vi "RecordDuringSaveSample_modified.vi"() -> ()   [LabVIEW 2015]
panel:
  out "Status":string
  out "Mem Frame Info":T1={"Start"=0, "End"=0, "Trigger"=0, "TwoStageLowToHigh"=0, "TwoStageHighToLow"=0, "TwoStageTiming"=0, "Event"=[1, 1, 1, 1, 1, 1, 1, 1, 1, 1], "EventCount"=0, "RecordedFrames"=0} {"RecordedFrames" max=0; "EventCount" max=0}
  out "IsSaving":bool
  in  "Save File Name":string caption="Save File Name :"
  in  "Save Path Name":path caption="Save Path Name :"
  out "Information":T2 caption="Frame"
  out "IsRecording":bool
  in  "Command":bool
  out "Picture":picture
  out "ChildNo":u32=1
  out "DeviceNo":u32
  in  "Stop":bool
  out "Error_Out":T3
  out "Color Type":enum16{"MONO", "COLOR"}(ring)
  out "Resolution":cluster{"Width":u32, "Height":u32}
  # "_1.avi"
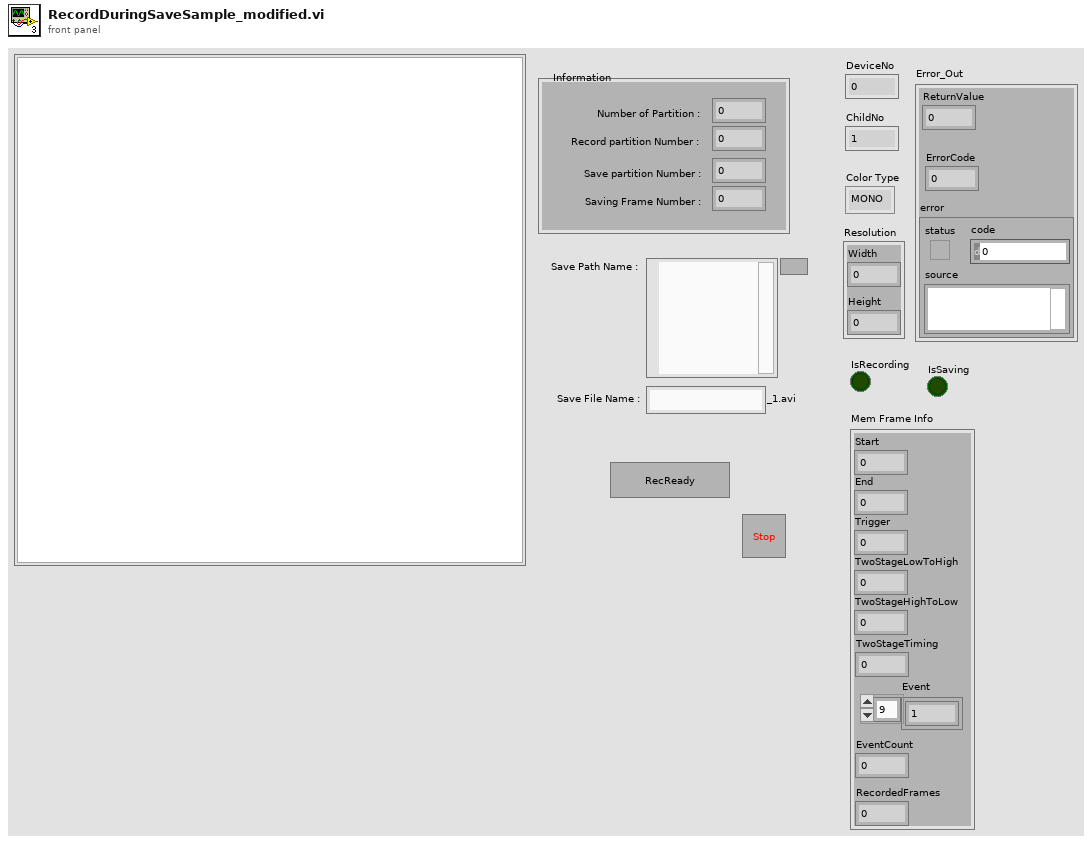
[diagram p1: front panel]
types:
  T1 = cluster{"Start":i32, "End":i32, "Trigger":i32, "TwoStageLowToHigh":i32, "TwoStageHighToLow":i32, "TwoStageTiming":u32, "Event":i32[], "EventCount":u32, "RecordedFrames":u32}
  T2 = cluster{"Number of Partition":u32, "Save Partition Number":u32, "Record Partition Number":u32, "Saving Frame Number":i32}
  T3 = cluster{"ReturnValue":u32, "ErrorCode":u32, "error ":errorcluster}
  T4 = enum16{"Initialize", "Device Initialize", "Status Check", "Save Image Open", "Save Image", "Save Image Close", "Update Window", "Default", "Exit", "Error"}
  T5 = typedef "LVBoundsTypeDef.ctl" = cluster{"Width":u32, "Height":u32}
  T6 = cluster{"Number of Partition":u32, "Save Partition Number":u32, "t":u32, "Saving Frame Number":i32}
  T7 = cluster{"Number of Partition":u32, "Save Partition Number":u32, "Record Partition Number":u32, i32}
  T8 = cluster{"Number of Partition":u32, "t":u32, "Record Partition Number":u32, "Saving Frame Number":i32}
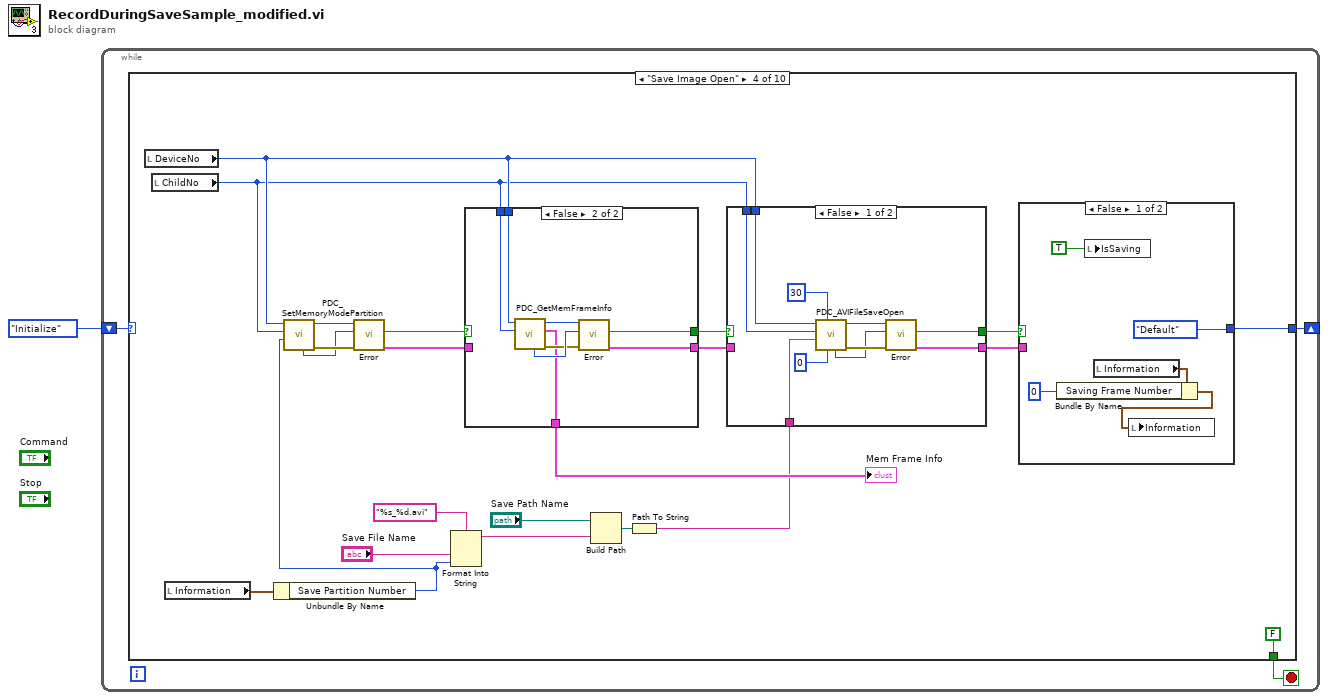
[diagram p0: block diagram]
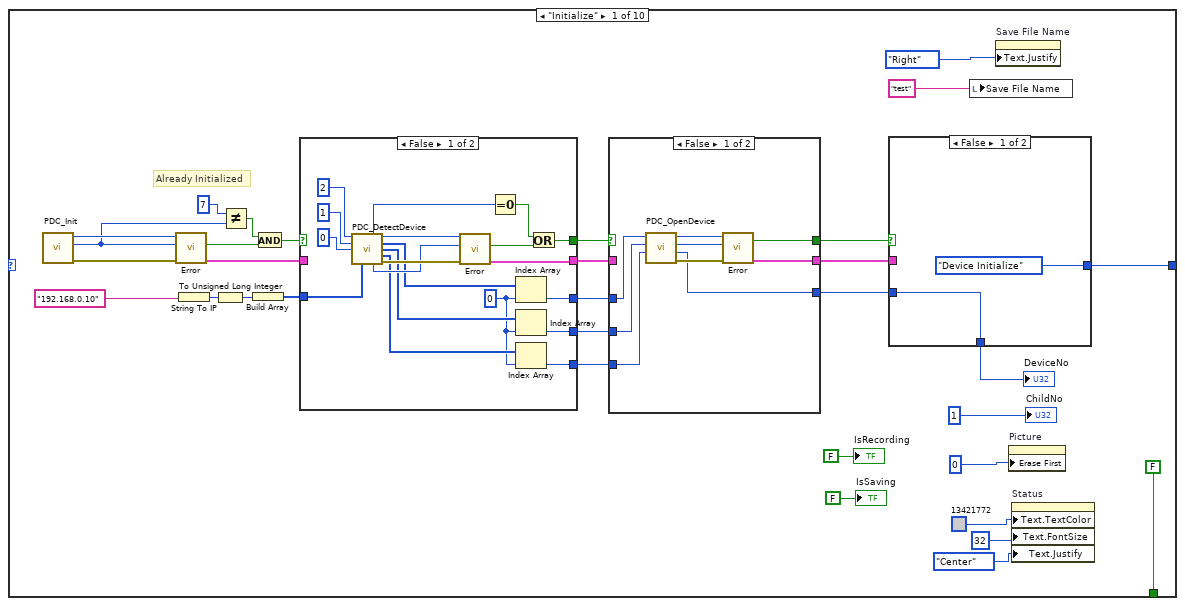
[diagram p2: hidden frame]
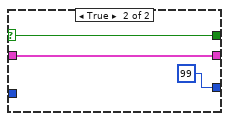
[diagram p3: hidden frame]
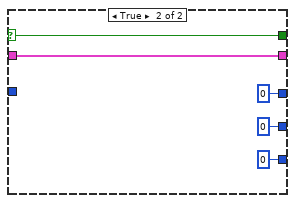
[diagram p4: hidden frame]
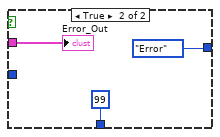
[diagram p5: hidden frame]
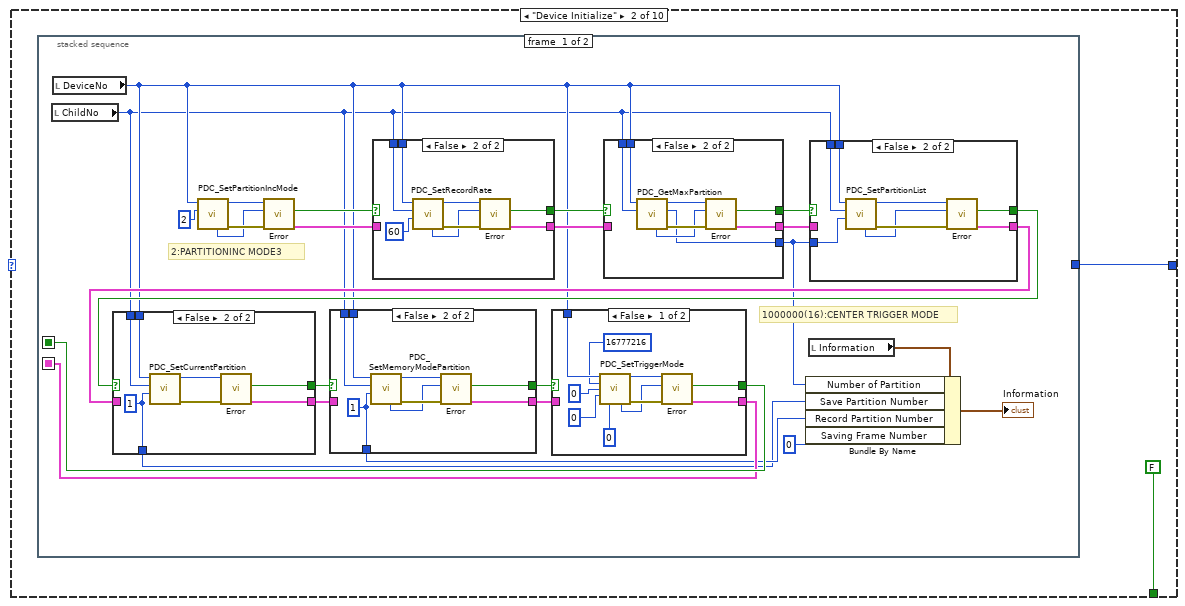
[diagram p6: hidden frame]
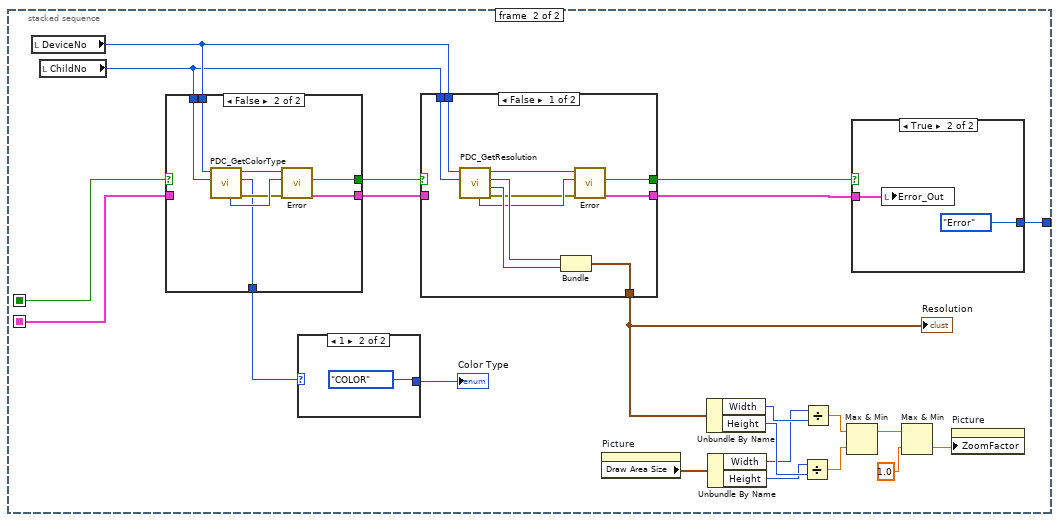
[diagram p13: hidden frame]
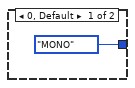
[diagram p16: hidden frame]
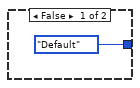
[diagram p17: hidden frame]
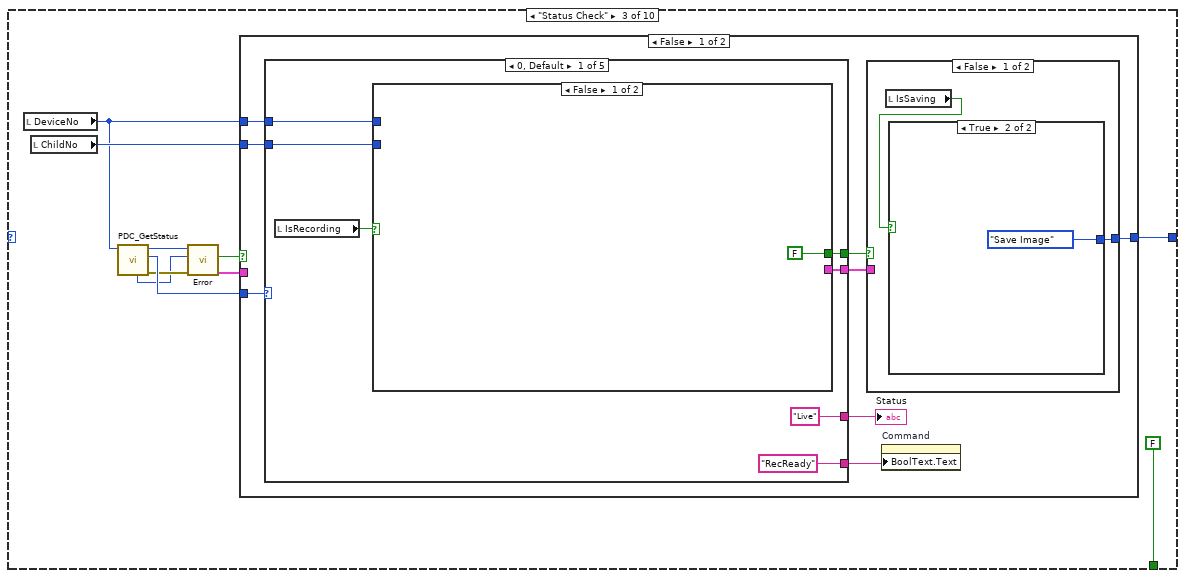
[diagram p18: hidden frame]
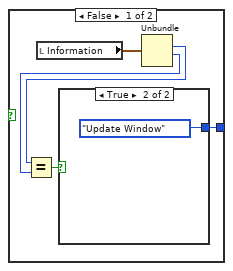
[diagram p19: hidden frame]
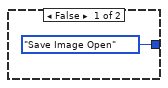
[diagram p20: hidden frame]
diagram:
  n1 = while {
    shift-right: [w2] -> _
    shift-left: T4."Initialize" ("Mode") -> [w3]
    stop <- w4 stop-if-true
    n2 = case shown="\"Save Image Open\"" w3 {
      tunnel: [FALSE FALSE FALSE FALSE FALSE FALSE FALSE FALSE TRUE FALSE] -> w4
      tunnel: [w15 w78 w216 w299 w343 w378 w405 w438 _ T4."Exit" ("Mode")] -> w2
      frame "Initialize" {
        # "Already Initialized"
        n3 = call "PDC_Init.vi"() -> ("error out"=w36:errorcluster, "ErrorCode"=w32:u32, "ReturnValue"=w35:u32)  [unwired: 9 in]
        n4 = call "Error.vi"("error in (no error)"=w36, "ErrorCode"=w32, "ReturnValue"=w35) -> ("Error_Out"=w29:T3, "Error?"=w34:bool)  [unwired: 7 in]
        n5 = String To IP(1:"192.168.0.10") -> (0:w22:u32)
        n6 = To Unsigned Long Integer(number=w22) -> (unsigned 32bit integer=w23:u32)
        n7 = Not Equal?(x=u32 7, y=w32) -> (x != y?=w33:bool)
        n8 = Build Array(w23) -> (w20:u32[])
        n9 = And(x=w33, y=w34) -> (x .and. y?=w30:bool)
        n10 = case shown="False" w30 {
          selector: w30 -> [_ w71]
          tunnel: w29 -> [_ w72]
          tunnel: [w59 w72] -> w27
          tunnel: [w61 w71] -> w28
          tunnel: w20 -> [w56 _]
          tunnel: [w51 u32 0 ("m_nDeviceCode")] -> w19
          tunnel: [w50 u32 0 ("m_nTmpDeviceNo")] -> w18
          tunnel: [w49 u32 0] -> w17
          frame False {
            w52 = 0 ("指標")
            n11 = call "PDC_DetectDevice.vi"("InterfaceCode"=u32 2, "DetectNum"=u32 1, "DetectParam"=u32 0, "DetectNo"=w56) -> ("DeviceNum"=w57:u32, "ReturnValue"=w63:u32, "DeviceCode"=w55:u32[], "TmpDeviceNo"=w54:u32[], "InterfaceCode(out)"=w53:u32[], "ErrorCode"=w62:u32, "error out"=w64:errorcluster)  [unwired: 5 in]
            n12 = call "Error.vi"("error in (no error)"=w64, "ErrorCode"=w62, "ReturnValue"=w63) -> ("Error_Out"=w59:T3, "Error?"=w60:bool)  [unwired: 7 in]
            n13 = Equal To 0?(x=w57) -> (x = 0?=w58:bool)
            n14 = Index Array(array=w55, index=w52) -> (element=w51:u32)
            n15 = Index Array(array=w54, index=w52) -> (element=w50:u32)
            n16 = Index Array(array=w53, index=w52) -> (element=w49:u32)
            n17 = Or(x=w58, y=w60) -> (x .or. y?=w61:bool)
          }
          frame True {
          }
        }
        n18 = case shown="False" w28 {
          selector: w28 -> [_ w47]
          tunnel: w27 -> [_ w48]
          tunnel: [w45 w48] -> w24
          tunnel: [w38 w47] -> w25
          tunnel: w19 -> [w39 _]
          tunnel: w18 -> [w40 _]
          tunnel: w17 -> [w41 _]
          tunnel: [w37 u32 99 ("DeviceNo")] -> w16
          frame False {
            n19 = call "PDC_OpenDevice.vi"("InterfaceCode"=w41, "TmpDeviceNo"=w40, "DeviceCode"=w39) -> ("error out"=w44:errorcluster, "DeviceNo"=w37:u32, "ErrorCode"=w42:u32, "ReturnValue"=w43:u32)  [unwired: 5 in]
            n20 = call "Error.vi"("error in (no error)"=w44, "ErrorCode"=w42, "ReturnValue"=w43) -> ("Error_Out"=w45:T3, "Error?"=w38:bool)  [unwired: 7 in]
          }
          frame True {
          }
        }
        n21 = case shown="False" w25 {
          tunnel: [T4."Device Initialize" ("Mode") T4."Error" ("Mode")] -> w15
          tunnel: w24 -> [_ w76]
          tunnel: w16 -> [w74 _]
          tunnel: [w74 u32 99 ("DeviceNo")] -> w12
          frame False {
          }
          frame True {
            "Error_Out" <- w76
          }
        }
        "DeviceNo" <- w12
        n22 = local write "Save File Name"("test" ("Save File Name")) -> ()
        n23 = property on="Save File Name" class="Str"("Text.Justify"=enum16{"Left", "Center", "Right"}."Right" ("テキスト.位置調整")) -> ()  [unwired: 2 in, 2 out]
        n24 = property on="Picture" class="Pict"("Erase First"=u8 0 ("最初に削除")) -> ()  [unwired: 2 in, 2 out]
        n25 = property on="Status" class="Str"("Text.TextColor"=u32 13421772, "Text.FontSize"=u32 32 ("テキスト.フォント:サイズ"), "Text.Justify"=enum16{"Left", "Center", "Right"}."Center" ("テキスト.位置調整")) -> ()  [unwired: 2 in, 2 out]
        "IsRecording" <- FALSE ("IsRecord")
        "ChildNo" <- u32 1
        "IsSaving" <- FALSE ("IsRecord")
      }
      frame "Device Initialize" {
        n26 = stacked-sequence {
          seq-local: [w88 _] -> [_ w181]
          seq-local: [w89 _] -> [_ w182]
          tunnel: [_ w178] -> w78
          frame #0 {
            # "1000000(16):CENTER TRIGGER MODE"
            # "2:PARTITIONINC MODE3"
            n27 = local read "ChildNo"() -> (w86:u32)
            n28 = local read "DeviceNo"() -> (w87:u32)
            n29 = call "PDC_SetPartitionIncMode.vi"("Mode"=u32 2, "DeviceNo"=w87) -> ("error out"=w104:errorcluster, "ReturnValue"=w105:u32, "ErrorCode"=w103:u32)  [unwired: 7 in]
            n30 = call "Error.vi"("error in (no error)"=w104, "ErrorCode"=w103, "ReturnValue"=w105) -> ("Error_Out"=w100:T3, "Error?"=w101:bool)  [unwired: 7 in]
            n31 = case shown="False" w101 {
              selector: w101 -> [w158 _]
              tunnel: w100 -> [w157 _]
              tunnel: [w157 w163] -> w99
              tunnel: [w158 w162] -> w98
              tunnel: w87 -> [_ w161]
              tunnel: w86 -> [_ w160]
              frame True {
              }
              frame False {
                n32 = call "PDC_SetRecordRate.vi"("Rate"=u32 60, "ChildNo"=w160, "DeviceNo"=w161) -> ("error out"=w165:errorcluster, "ReturnValue"=w166:u32, "ErrorCode"=w164:u32)  [unwired: 6 in]
                n33 = call "Error.vi"("error in (no error)"=w165, "ErrorCode"=w164, "ReturnValue"=w166) -> ("Error_Out"=w163:T3, "Error?"=w162:bool)  [unwired: 7 in]
              }
            }
            n34 = case shown="False" w98 {
              selector: w98 -> [w148 _]
              tunnel: w99 -> [w147 _]
              tunnel: [w148 w154] -> w97
              tunnel: [w147 w153] -> w96
              tunnel: w87 -> [_ w151]
              tunnel: w86 -> [_ w150]
              tunnel: [_ w149] -> w83
              frame True {
              }
              frame False {
                n35 = call "PDC_GetMaxPartition.vi"("ChildNo"=w150, "DeviceNo"=w151) -> ("error out"=w155:errorcluster, "Count"=w149:u32, "ReturnValue"=w156:u32, "ErrorCode"=w152:u32)  [unwired: 5 in, 1 out]
                n36 = call "Error.vi"("error in (no error)"=w155, "ErrorCode"=w152, "ReturnValue"=w156) -> ("Error_Out"=w153:T3, "Error?"=w154:bool)  [unwired: 7 in]
              }
            }
            n37 = local read "Information"() -> (w85:T2)
            n38 = case shown="False" w97 {
              selector: w97 -> [w138 _]
              tunnel: w96 -> [w137 _]
              tunnel: [w138 w143] -> w93
              tunnel: [w137 w142] -> w92
              tunnel: w87 -> [_ w141]
              tunnel: w86 -> [_ w140]
              tunnel: w83 -> [_ w139]
              frame True {
              }
              frame False {
                n39 = call "PDC_SetPartitionList.vi"("Count"=w139, "ChildNo"=w140, "DeviceNo"=w141) -> ("error out"=w146:errorcluster, "ReturnValue"=w145:u32, "ErrorCode"=w144:u32)  [unwired: 6 in]
                n40 = call "Error.vi"("error in (no error)"=w146, "ErrorCode"=w144, "ReturnValue"=w145) -> ("Error_Out"=w142:T3, "Error?"=w143:bool)  [unwired: 7 in]
              }
            }
            n41 = case shown="False" w93 {
              selector: w93 -> [w129 _]
              tunnel: [w129 w134] -> w95
              tunnel: [w128 w133] -> w94
              tunnel: w92 -> [w128 _]
              tunnel: w87 -> [_ w132]
              tunnel: w86 -> [_ w131]
              tunnel: [_ w130] -> w80
              frame True {
              }
              frame False {
                w130 = u32 1 ("No")
                n42 = call "PDC_SetCurrentPartition.vi"("No"=w130, "ChildNo"=w131, "DeviceNo"=w132) -> ("error out"=w135:errorcluster, "ReturnValue"=w136:u32)  [unwired: 6 in, 1 out]
                n43 = call "Error.vi"("error in (no error)"=w135, "ReturnValue"=w136) -> ("Error_Out"=w133:T3, "Error?"=w134:bool)  [unwired: 8 in]
              }
            }
            n44 = case shown="False" w95 {
              selector: w95 -> [w119 _]
              tunnel: w94 -> [w118 _]
              tunnel: [w119 w124] -> w91
              tunnel: [w118 w121] -> w90
              tunnel: w87 -> [_ w123]
              tunnel: w86 -> [_ w122]
              tunnel: [_ w120] -> w81
              frame True {
              }
              frame False {
                w120 = u32 1 ("No")
                n45 = call "PDC_SetMemoryModePartition.vi"("No"=w120, "ChildNo"=w122, "DeviceNo"=w123) -> ("error out"=w126:errorcluster, "ReturnValue"=w127:u32, "ErrorCode"=w125:u32)  [unwired: 6 in]
                n46 = call "Error.vi"("error in (no error)"=w126, "ErrorCode"=w125, "ReturnValue"=w127) -> ("Error_Out"=w121:T3, "Error?"=w124:bool)  [unwired: 7 in]
              }
            }
            n47 = case shown="False" w91 {
              selector: w91 -> [_ w117]
              tunnel: w90 -> [_ w116]
              tunnel: [w111 w117] -> w89
              tunnel: [w115 w116] -> w88
              tunnel: w87 -> [w110 _]
              frame False {
                n48 = call "PDC_SetTriggerMode.vi"("DeviceNo"=w110, "Mode"=u32 16777216, "AFrames"=u32 0, "RFrames"=u32 0, "RCount"=u32 0) -> ("ReturnValue"=w113:u32, "ErrorCode"=w112:u32, "error out"=w114:errorcluster)  [unwired: 8 in]
                n49 = call "Error.vi"("error in (no error)"=w114, "ErrorCode"=w112, "ReturnValue"=w113) -> ("Error_Out"=w115:T3, "Error?"=w111:bool)  [unwired: 7 in]
              }
              frame True {
              }
            }
            n50 = Bundle By Name(cluster=w85, "Number of Partition"=w83, "Save Partition Number"=w80, "Record Partition Number"=w81, "Saving Frame Number"=0) -> (→"Information":T2)
          }
          frame #1 {
            n51 = local read "DeviceNo"() -> (w180:u32)
            n52 = local read "ChildNo"() -> (w179:u32)
            n53 = case shown="False" w182 {
              selector: w182 -> [w190 _]
              tunnel: [_ w195] -> w188
              tunnel: [w190 w194] -> w186
              tunnel: [w189 w193] -> w185
              tunnel: w181 -> [w189 _]
              tunnel: w180 -> [_ w192]
              tunnel: w179 -> [_ w191]
              frame True {
              }
              frame False {
                n54 = call "PDC_GetColorType.vi"("ChildNo"=w191, "DeviceNo"=w192) -> ("error out"=w196:errorcluster, "Mode"=w195:i8, "ReturnValue"=w198:u32, "ErrorCode"=w197:u32)  [unwired: 6 in]
                n55 = call "Error.vi"("error in (no error)"=w196, "ErrorCode"=w197, "ReturnValue"=w198) -> ("Error_Out"=w193:T3, "Error?"=w194:bool)  [unwired: 7 in]
              }
            }
            n56 = case shown="1" w188 {
              tunnel: [enum16{"MONO", "COLOR"}."MONO" enum16{"MONO", "COLOR"}."COLOR"] -> w187
              frame 0, Default {
              }
              frame 1 {
              }
            }
            "Color Type" <- w187
            n57 = case shown="False" w186 {
              selector: w186 -> [_ w209]
              tunnel: w185 -> [_ w210]
              tunnel: [w202 w210] -> w183
              tunnel: [w203 w209] -> w184
              tunnel: [w201 _] -> w176
              tunnel: w180 -> [w200 _]
              tunnel: w179 -> [w199 _]
              frame False {
                n58 = call "PDC_GetResolution.vi"("ChildNo"=w199, "DeviceNo"=w200) -> ("error out"=w205:errorcluster, "Height"=w208:u32, "Width"=w207:u32, "ReturnValue"=w204:u32, "ErrorCode"=w206:u32)  [unwired: 5 in]
                n59 = Bundle("Width"=w207, "Height"=w208) -> (w201:cluster{"Width":u32, "Height":u32})  [unwired: 1 in]
                n60 = call "Error.vi"("error in (no error)"=w205, "ErrorCode"=w206, "ReturnValue"=w204) -> ("Error_Out"=w202:T3, "Error?"=w203:bool)  [unwired: 7 in]
              }
              frame True {
              }
            }
            "Resolution" <- w176
            n61 = property on="Picture" class="Pict"() -> ("Draw Area Size"=w177:T5)  [unwired: 2 in, 2 out]
            n62 = Unbundle By Name(w176) -> ("Width"=w175:u32, "Height"=w174:u32)
            n63 = Unbundle By Name(w177) -> ("Width"=w173:u32, "Height"=w172:u32)
            n64 = Divide(x=w172, y=w174) -> (x/y=w170:dbl)
            n65 = Divide(x=w173, y=w175) -> (x/y=w171:dbl)
            n66 = Max & Min(x=w171, y=w170) -> (max(x,y)=w169:dbl)  [unwired: 1 out]
            n67 = case shown="True" w184 {
              tunnel: [T4."Default" ("Mode") T4."Error" ("Mode")] -> w178
              tunnel: w183 -> [_ w215]
              frame False {
              }
              frame True {
                n68 = local write "Error_Out"(w215) -> ()
              }
            }
            n69 = Max & Min(x=w169, y=1.0) -> (min(x,y)=w168:dbl)  [unwired: 1 out]
            n70 = property on="Picture" class="Pict"("ZoomFactor"=w168) -> ()  [unwired: 2 in, 2 out]
          }
        }
      }
      frame "Status Check" {
        n71 = local read "DeviceNo"() -> (w220:u32)
        n72 = local read "ChildNo"() -> (w221:u32)
        n73 = call "PDC_GetStatus.vi"("DeviceNo"=w220) -> ("error out"=w219:errorcluster, "Status"=w222:u32, "ReturnValue"=w218:u32, "ErrorCode"=w217:u32)  [unwired: 7 in]
        n74 = call "Error.vi"("error in (no error)"=w219, "ErrorCode"=w217, "ReturnValue"=w218) -> ("Error_Out"=w223:T3, "Error?"=w224:bool)  [unwired: 7 in]
        n75 = case shown="False" w224 {
          tunnel: w223 -> [_ w281]
          tunnel: w222 -> [w233 _]
          tunnel: w220 -> [w232 _]
          tunnel: w221 -> [w231 _]
          tunnel: [w227 T4."Error" ("Mode")] -> w216
          frame False {
            n76 = case shown="0, Default" w233 {
              tunnel: w232 -> [w251 _ _ _ _]
              tunnel: w231 -> [w250 _ _ _ _]
              tunnel: ["Live" "PlayBack" "RecReady" "Endless" "Record"] -> w226
              tunnel: ["RecReady" "Live" "Trigger In" "Trigger In" "Cancel"] -> w230
              tunnel: [w247 _ _ _ _] -> w229
              tunnel: [w246 _ _ _ _] -> w228
              frame 0, Default {
                n77 = local read "IsRecording"() -> (w252:bool)
                n78 = case shown="False" w252 {
                  tunnel: w251 -> [_ w259]
                  tunnel: w250 -> [_ w258]
                  tunnel: [FALSE ("Error?") w257] -> w247
                  tunnel: [_ w256] -> w246
                  frame False {
                  }
                  frame True {
                    n79 = local read "Information"() -> (w267:T2)
                    n80 = local write "IsRecording"(FALSE ("IsRecord")) -> ()
                    n81 = Unbundle(w267) -> ("Number of Partition"=w263:u32, "Save Partition Number"=w255:u32, "Record Partition Number"=w266:u32, "Saving Frame Number"=w264:i32)
                    n82 = Equal?(x=w263, y=w266) -> (x = y?=w270:bool)
                    n83 = Increment(x=w266) -> (x+1=w268:u32)
                    n84 = Select(t=u32 1, s=w270, f=w268) -> (s? t:f=w254:u32)
                    n85 = call "PDC_SetCurrentPartition.vi"("No"=w254, "ChildNo"=w258, "DeviceNo"=w259) -> ("error out"=w262:errorcluster, "ReturnValue"=w261:u32, "ErrorCode"=w260:u32)  [unwired: 6 in]
                    n86 = call "Error.vi"("error in (no error)"=w262, "ErrorCode"=w260, "ReturnValue"=w261) -> ("Error_Out"=w256:T3, "Error?"=w257:bool)  [unwired: 7 in]
                    n87 = Bundle("Number of Partition"=w263, "Save Partition Number"=w255, "t"=w254, "Saving Frame Number"=w264) -> (w265:T6)  [unwired: 1 in]
                    n88 = local write "Information"(w265) -> ()
                  }
                }
              }
              frame 1 {
              }
              frame 2 {
              }
              frame 4 {
              }
              frame 8 {
              }
            }
            "Status" <- w226
            n89 = case shown="False" w229 {
              tunnel: w228 -> [_ w245]
              tunnel: [w234 T4."Error" ("Mode")] -> w227
              frame False {
                n90 = local read "IsSaving"() -> (w235:bool)
                n91 = case shown="True" w235 {
                  tunnel: [w236 T4."Save Image" ("Mode")] -> w234
                  frame False {
                    n92 = local read "Information"() -> (w240:T2)
                    n93 = Unbundle(w240) -> ("Save Partition Number"=w237:u32, "Record Partition Number"=w238:u32)  [unwired: 2 out]
                    n94 = Equal?(x=w237, y=w238) -> (x = y?=w239:bool)
                    n95 = case shown="True" w239 {
                      tunnel: [T4."Save Image Open" ("Mode") T4."Update Window" ("Mode")] -> w236
                      frame False {
                      }
                      frame True {
                      }
                    }
                  }
                  frame True {
                  }
                }
              }
              frame True {
                n96 = local write "Error_Out"(w245) -> ()
              }
            }
            n97 = property on="Command" class="Bool (strict)"("BoolText.Text"=w230) -> ()  [unwired: 2 in, 2 out]
          }
          frame True {
            n98 = local write "Error_Out"(w281) -> ()
          }
        }
      }
      frame "Save Image Open" {
        n99 = local read "DeviceNo"() -> (w286:u32)
        n100 = local read "ChildNo"() -> (w285:u32)
        n101 = local read "Information"() -> (w292:T2)
        n102 = Unbundle By Name(w292) -> ("Save Partition Number"=w282:u32)
        n103 = call "PDC_SetMemoryModePartition.vi"("No"=w282, "ChildNo"=w285, "DeviceNo"=w286) -> ("error out"=w288:errorcluster, "ReturnValue"=w289:u32, "ErrorCode"=w287:u32)  [unwired: 6 in]
        n104 = call "Error.vi"("error in (no error)"=w288, "ErrorCode"=w287, "ReturnValue"=w289) -> ("Error_Out"=w283:T3, "Error?"=w284:bool)  [unwired: 7 in]
        n105 = Format Into String(format string="%s_%d.avi" ("形式文字列"), "Save File Name", w282) -> (resulting string=w291:string)  [unwired: 2 in, 1 out]
        n106 = case shown="False" w284 {
          selector: w284 -> [w305 _]
          tunnel: [w305 w310] -> w303
          tunnel: [w304 w309] -> w302
          tunnel: w286 -> [_ w308]
          tunnel: w285 -> [_ w307]
          tunnel: [_ w306] -> w298
          tunnel: w283 -> [w304 _]
          frame True {
          }
          frame False {
            n107 = call "PDC_GetMemFrameInfo.vi"("ChildNo"=w307, "DeviceNo"=w308) -> ("error out"=w311:errorcluster, "Frame"=w306:T1, "ReturnValue"=w312:u32, "ErrorCode"=w313:u32)  [unwired: 6 in]
            n108 = call "Error.vi"("error in (no error)"=w311, "ErrorCode"=w313, "ReturnValue"=w312) -> ("Error_Out"=w309:T3, "Error?"=w310:bool)  [unwired: 7 in]
          }
        }
        "Mem Frame Info" <- w298
        n109 = Build Path(base path="Save Path Name", name or relative path=w291) -> (appended path=w295:path)
        n110 = Path To String(path=w295) -> (string=w290:string)
        n111 = case shown="False" w303 {
          selector: w303 -> [_ w332]
          tunnel: w302 -> [_ w331]
          tunnel: [w329 w332] -> w301
          tunnel: [w330 w331] -> w300
          tunnel: w286 -> [w324 _]
          tunnel: w285 -> [w323 _]
          tunnel: w290 -> [w325 _]
          frame False {
            n112 = call "PDC_AVIFileSaveOpen.vi"("ShowCompressDlg"=u32 0, "Rate"=30, "FileName"=w325, "ChildNo"=w323, "DeviceNo"=w324) -> ("error out"=w327:errorcluster, "ReturnValue"=w328:u32, "ErrorCode"=w326:u32)  [unwired: 4 in]
            n113 = call "Error.vi"("error in (no error)"=w327, "ErrorCode"=w326, "ReturnValue"=w328) -> ("Error_Out"=w330:T3, "Error?"=w329:bool)  [unwired: 7 in]
          }
          frame True {
          }
        }
        n114 = case shown="False" w301 {
          tunnel: w300 -> [_ w320]
          tunnel: [T4."Default" ("Mode") T4."Error" ("Mode")] -> w299
          frame False {
            n115 = local write "IsSaving"(TRUE) -> ()
            n116 = local read "Information"() -> (w315:T2)
            n117 = Bundle By Name(cluster=w315, "Saving Frame Number"=0) -> (w314:T2)
            n118 = local write "Information"(w314) -> ()
          }
          frame True {
            n119 = local write "Error_Out"(w320) -> ()
          }
        }
      }
      frame "Save Image" {
        n120 = local read "Mem Frame Info"() -> (w355:T1)
        n121 = local read "Information"() -> (w356:T2)
        n122 = Unbundle(w356) -> ("Number of Partition"=w350:u32, "Save Partition Number"=w349:u32, "Record Partition Number"=w348:u32, "Saving Frame Number"=w347:i32)
        n123 = Unbundle By Name(w355) -> ("RecordedFrames"=w335:u32, "Start"=w351:i32, "End"=w352:i32)
        n124 = Add(x=w351, y=w347) -> (x+y=w354:i32)
        n125 = Increment(x=w347) -> (x+1=w334:i32)
        n126 = Less Than 0?(x=w354) -> (x < 0?=w353:bool)
        n127 = case shown="False" w353 {
          tunnel: w354 -> [w364 w367]
          tunnel: [w364 w365] -> w337
          tunnel: w352 -> [_ w368]
          tunnel: w351 -> [_ w370]
          frame False {
          }
          frame True {
            n128 = Absolute Value(x=w370) -> (abs(x)=w369:i32)
            n129 = Compound Arithmetic op=ADD(w369, w368, w367, 1 ("値")) -> (w365:i32)
          }
        }
        n130 = local read "DeviceNo"() -> (w339:u32)
        n131 = local read "ChildNo"() -> (w338:u32)
        n132 = Bundle("Number of Partition"=w350, "Save Partition Number"=w349, "Record Partition Number"=w348, w334) -> (w346:T7)  [unwired: 1 in]
        n133 = local write "Information"(w346) -> ()
        n134 = call "PDC_AVIFileSave.vi"("FrameNo"=w337, "ChildNo"=w338, "DeviceNo"=w339) -> ("error out"=w341:errorcluster, "ReturnValue"=w342:u32, "ErrorCode"=w340:u32)  [unwired: 5 in, 1 out]
        n135 = To Unsigned Long Integer(number=w334) -> (unsigned 32bit integer=w333:u32)
        n136 = call "Error.vi"("error in (no error)"=w341, "ErrorCode"=w340, "ReturnValue"=w342) -> ("Error_Out"=w344:T3, "Error?"=w345:bool)  [unwired: 7 in]
        n137 = Equal?(x=w335, y=w333) -> (x = y?=w336:bool)
        n138 = case shown="False" w345 {
          tunnel: w344 -> [_ w363]
          tunnel: [w359 T4."Save Image Close" ("Mode")] -> w343
          tunnel: w336 -> [w358 _]
          frame False {
            n139 = case shown="False" w358 {
              tunnel: [T4."Update Window" ("Mode") T4."Save Image Close" ("Mode")] -> w359
              frame False {
              }
              frame True {
              }
            }
          }
          frame True {
            n140 = local write "Error_Out"(w363) -> ()
          }
        }
      }
      frame "Save Image Close" {
        n141 = local read "DeviceNo"() -> (w372:u32)
        n142 = local read "ChildNo"() -> (w371:u32)
        n143 = call "PDC_AVIFileSaveClose.vi"("ChildNo"=w371, "DeviceNo"=w372) -> ("error out"=w375:errorcluster, "ReturnValue"=w374:u32, "ErrorCode"=w373:u32)  [unwired: 7 in]
        n144 = call "Error.vi"("error in (no error)"=w375, "ErrorCode"=w373, "ReturnValue"=w374) -> ("Error_Out"=w381:T3, "Error?"=w382:bool)  [unwired: 7 in]
        n145 = case shown="False" w382 {
          selector: w382 -> [_ w404]
          tunnel: w381 -> [_ w403]
          tunnel: [w393 w404] -> w380
          tunnel: [w392 w403] -> w379
          tunnel: w372 -> [w387 _]
          tunnel: w371 -> [w386 _]
          frame False {
            n146 = local read "Information"() -> (w402:T2)
            n147 = Unbundle(w402) -> ("Number of Partition"=w397:u32, "Save Partition Number"=w395:u32, "Record Partition Number"=w399:u32, "Saving Frame Number"=w400:i32)
            n148 = Equal?(x=w397, y=w395) -> (x = y?=w398:bool)
            n149 = Increment(x=w395) -> (x+1=w396:u32)
            n150 = Select(t=u32 1, s=w398, f=w396) -> (s? t:f=w388:u32)
            n151 = call "PDC_SetMemoryModePartition.vi"("No"=w388, "ChildNo"=w386, "DeviceNo"=w387) -> ("error out"=w390:errorcluster, "ReturnValue"=w391:u32, "ErrorCode"=w389:u32)  [unwired: 6 in]
            n152 = call "Error.vi"("error in (no error)"=w390, "ErrorCode"=w389, "ReturnValue"=w391) -> ("Error_Out"=w392:T3, "Error?"=w393:bool)  [unwired: 7 in]
            n153 = Bundle("Number of Partition"=w397, "t"=w388, "Record Partition Number"=w399, "Saving Frame Number"=w400) -> (w401:T8)  [unwired: 1 in]
            n154 = local write "Information"(w401) -> ()
          }
          frame True {
          }
        }
        n155 = case shown="False" w380 {
          tunnel: w379 -> [_ w385]
          tunnel: [T4."Default" ("Mode") T4."Error" ("Mode")] -> w378
          frame False {
          }
          frame True {
            n156 = local write "Error_Out"(w385) -> ()
          }
        }
        n157 = local write "IsSaving"(FALSE ("IsSaving")) -> ()
      }
      frame "Update Window" {
        n158 = local read "Information"() -> (w416:T2)
        n159 = Unbundle By Name(w416) -> ("Saving Frame Number"=w415:i32)
        n160 = local read "IsSaving"() -> (w412:bool)
        n161 = local read "Color Type"() -> (w409:enum16{"MONO", "COLOR"})
        n162 = local read "Resolution"() -> (w408:cluster{"Width":u32, "Height":u32})
        n163 = local read "DeviceNo"() -> (w411:u32)
        n164 = local read "ChildNo"() -> (w410:u32)
        n165 = Quotient & Remainder(x=w415, y=8) -> (x-y*floor(x/y)=w407:i32)  [unwired: 1 out]
        n166 = Not Equal To 0?(x=w407) -> (x != 0?=w406:bool)
        n167 = And(x=w412, y=w406) -> (x .and. y?=w413:bool)
        n168 = case shown="False" w413 {
          tunnel: w411 -> [_ w426]
          tunnel: w410 -> [_ w425]
          tunnel: w409 -> [_ w421]
          tunnel: w408 -> [_ w420]
          tunnel: [T4."Default" ("Mode") w422] -> w405
          frame True {
          }
          frame False {
            n169 = call "PDC_GetLiveImageData.vi"("Resolution"=w420, "ColorType"=w421, "BitDepth"=u32 8, "ChildNo"=w425, "DeviceNo"=w426) -> ("error out"=w427:errorcluster, "ErrorCode"=w429:u32, "ReturnValue"=w428:u32, "Data(8Bit)"=w419:u8[])  [unwired: 2 in, 1 out]
            n170 = call "Error.vi"("error in (no error)"=w427, "ErrorCode"=w429, "ReturnValue"=w428) -> ("Error_Out"=w423:T3, "Error?"=w424:bool)  [unwired: 7 in]
            n171 = case shown="False" w424 {
              tunnel: [T4."Error" ("Mode") T4."Default" ("Mode")] -> w422
              tunnel: w423 -> [w431 _]
              tunnel: w421 -> [_ w435]
              tunnel: w420 -> [_ w434]
              tunnel: w419 -> [_ w433]
              frame True {
                n172 = local write "Error_Out"(w431) -> ()
              }
              frame False {
                n173 = call "GetPictureData.vi"("Resolution"=w434, "Data(8Bit)"=w433, "ColorType"=w435) -> ("new picture"=→"Picture":picture)  [unwired: 4 in]
              }
            }
          }
        }
      }
      frame "Default", Default {
        n174 = event shown="[0] Timeout" {
          selector: _ -> [_ _ _]
          dyn-events: _ -> [_ _ _]
          timeout: 1 -> [_ _ _]
          tunnel: [T4."Status Check" ("Mode") w442 T4."Exit" ("Mode")] -> w438
          event Timeout {
            n175 = event-data() -> ()  [unwired: 1 in, 2 out]
          }
          event "Command": Value Change {
            n176 = event-data() -> ("NewVal"=w443:bool)  [unwired: 1 in, 4 out]
            n177 = case shown="True" w443 {
              tunnel: [T4."Default" ("Mode") w446] -> w442
              frame False {
              }
              frame True {
                n178 = local read "DeviceNo"() -> (w445:u32)
                n179 = call "PDC_GetStatus.vi"("DeviceNo"=w445) -> ("error out"=w454:errorcluster, "Status"=w449:u32, "ReturnValue"=w453:u32, "ErrorCode"=w452:u32)  [unwired: 7 in]
                n180 = call "Error.vi"("error in (no error)"=w454, "ErrorCode"=w452, "ReturnValue"=w453) -> ("Error_Out"=w450:T3, "Error?"=w451:bool)  [unwired: 7 in]
                n181 = case shown="False" w451 {
                  selector: w451 -> [_ w496]
                  tunnel: w450 -> [_ w497]
                  tunnel: [w459 w497] -> w447
                  tunnel: [w458 w496] -> w448
                  tunnel: w449 -> [w461 _]
                  tunnel: w445 -> [w460 _]
                  frame False {
                    n182 = case shown="8" w461 {
                      tunnel: w460 -> [w462 w470 w476 w483 w491]
                      tunnel: [w467 w474 w481 w488 w495] -> w459
                      tunnel: [w466 w473 w480 w487 w494] -> w458
                      frame 0, Default {
                        n183 = call "PDC_SetRecReady.vi"("DeviceNo"=w462) -> ("error out"=w465:errorcluster, "ReturnValue"=w464:u32, "ErrorCode"=w463:u32)  [unwired: 8 in]
                        n184 = call "Error.vi"("error in (no error)"=w465, "ErrorCode"=w463, "ReturnValue"=w464) -> ("Error_Out"=w467:T3, "Error?"=w466:bool)  [unwired: 7 in]
                      }
                      frame 1 {
                        n185 = call "PDC_SetStatus.vi"("Mode"=u32 0, "DeviceNo"=w470) -> ("error out"=w472:errorcluster, "ReturnValue"=w471:u32, "ErrorCode"=w469:u32)  [unwired: 7 in]
                        n186 = call "Error.vi"("error in (no error)"=w472, "ErrorCode"=w469, "ReturnValue"=w471) -> ("Error_Out"=w474:T3, "Error?"=w473:bool)  [unwired: 7 in]
                      }
                      frame 2 {
                        n187 = call "PDC_TriggerIn.vi"("DeviceNo"=w476) -> ("error out"=w479:errorcluster, "ReturnValue"=w478:u32, "ErrorCode"=w477:u32)  [unwired: 8 in]
                        n188 = call "Error.vi"("error in (no error)"=w479, "ErrorCode"=w477, "ReturnValue"=w478) -> ("Error_Out"=w481:T3, "Error?"=w480:bool)  [unwired: 7 in]
                        n189 = local write "IsRecording"(TRUE ("IsRecord")) -> ()
                      }
                      frame 4 {
                        n190 = call "PDC_TriggerIn.vi"("DeviceNo"=w483) -> ("error out"=w486:errorcluster, "ReturnValue"=w485:u32, "ErrorCode"=w484:u32)  [unwired: 8 in]
                        n191 = call "Error.vi"("error in (no error)"=w486, "ErrorCode"=w484, "ReturnValue"=w485) -> ("Error_Out"=w488:T3, "Error?"=w487:bool)  [unwired: 7 in]
                        n192 = local write "IsRecording"(TRUE ("IsRecord")) -> ()
                      }
                      frame 8 {
                        n193 = call "PDC_SetStatus.vi"("Mode"=u32 0, "DeviceNo"=w491) -> ("error out"=w493:errorcluster, "ReturnValue"=w492:u32, "ErrorCode"=w490:u32)  [unwired: 7 in]
                        n194 = call "Error.vi"("error in (no error)"=w493, "ErrorCode"=w490, "ReturnValue"=w492) -> ("Error_Out"=w495:T3, "Error?"=w494:bool)  [unwired: 7 in]
                      }
                    }
                  }
                  frame True {
                  }
                }
                n195 = case shown="False" w448 {
                  tunnel: w447 -> [_ w457]
                  tunnel: [T4."Default" ("Mode") T4."Error" ("Mode")] -> w446
                  frame False {
                  }
                  frame True {
                    n196 = local write "Error_Out"(w457) -> ()
                  }
                }
              }
            }
          }
          event "Stop": Value Change {
            n197 = event-data() -> ()  [unwired: 1 in, 5 out]
          }
        }
      }
      frame "Exit" {
        n198 = local read "DeviceNo"() -> (w499:u32)
        n199 = case shown="Default" w499 {
          selector: w499 -> [_ w501]
          frame 99 {
          }
          frame Default {
            n200 = call "PDC_CloseDevice.vi"("DeviceNo"=w501) -> ()  [unwired: 8 in, 3 out]
          }
        }
      }
      frame "Error" {
        w505 = "\r\n"
        n201 = local read "Error_Out"() -> (w503:T3)
        n202 = Unbundle By Name(w503) -> ("error"=w520:errorcluster, "error.source"=w517:string, "error.code"=w516:i32, "ReturnValue"=w513:u32, "ErrorCode"=w512:u32)
        n203 = Number To Decimal String(number=w516) -> (decimal integer string=w514:string)  [unwired: 1 out]
        n204 = Number To Decimal String(number=w513) -> (decimal integer string=w510:string)  [unwired: 1 out]
        n205 = Number To Decimal String(number=w512) -> (decimal integer string=w508:string)  [unwired: 1 out]
        n206 = call <vilib>:"Clear Errors.vi"("error in (no error)"=w520) -> ("error out"=w519:errorcluster)  [unwired: 1 in, 5 out]
        n207 = Concatenate Strings("<<Error !!>>", w505, w505, w505, "Source=", w517, w505, "LabError=", w514, w505, "ReturnType=", w510, w505, "ErrorCode=", w508) -> (w507:string)
        n208 = call "メッセージ表示"("error in (no error)"=w519, "Message"=w507) -> ()  [unwired: 1 in, 9 out]
      }
    }
  }
